vi "Identify.vi"(3 "error in":errorcluster, 5 "VISA arduino in":refnum<visa-resource-name>) -> (0 "error out":errorcluster, 1 "identification":string, 2 "VISA arduino out":refnum<visa-resource-name>)   [LabVIEW 2021]
uses:
  <vilib>/Utility/error.llb/Error Cluster From Error Code.vi
  <vilib>/ErrorRing/Error Ring.xnode
panel:
  out "delay":u32
  # "Private"
  # "Public"
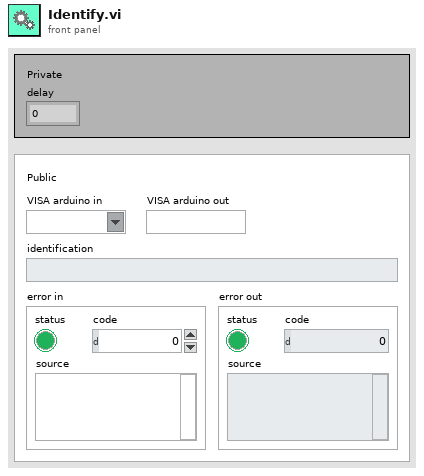
[diagram p1: front panel]
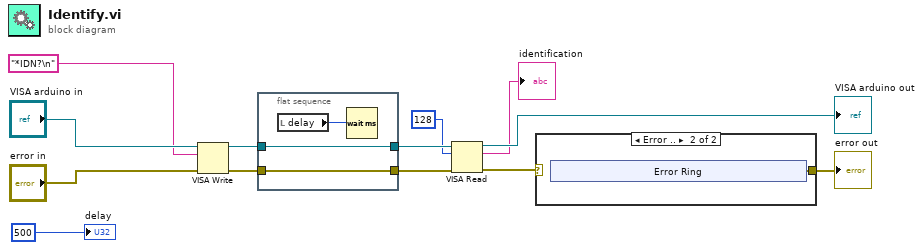
[diagram p0: block diagram]
diagram:
  n1 = VISA Write(VISA resource name="VISA arduino in", write buffer="*IDN?\n", error in (no error)="error in") -> (VISA resource name out=w12:refnum<visa-resource-name>, error out=w11:errorcluster)  [unwired: 1 out]
  n2 = flat-sequence {
    tunnel: [w16] -> w5
    tunnel: w12 -> [w16]
    tunnel: [w15] -> w6
    tunnel: w11 -> [w15]
    frame #0 {
      n3 = local read "delay"() -> (w14:u32)
      n4 = Wait (ms)(milliseconds to wait=w14) -> ()  [unwired: 1 out]
    }
  }
  n5 = VISA Read(VISA resource name=w5, byte count=u32 128, error in (no error)=w6) -> (VISA resource name out=→"VISA arduino out":refnum<visa-resource-name>, read buffer=→"identification":string, error out=w3:errorcluster)  [unwired: 1 out]
  n6 = case shown="Error .." w3 {
    selector: w3 -> [w17 _]
    tunnel: [w17 w18] -> w10
    frame No Error {
    }
    frame Error {
      n7 = xnode "Error Ring"() -> ("error out"=w18:errorcluster)
    }
  }
  "error out" <- w10
  "delay" <- u32 500
